vi "FilePath.vi"(8 "error in":errorcluster) -> (0 "error out":errorcluster, 3 "File path":path)   [LabVIEW 2016]
doc: "This SubVI designed for create filepath\nwith specific filename for saving picture\nto local disc. File name generate following\nto current date/time"
panel:
  # "This SubVI designed for create filepath\nwith specific filename for saving picture\nto local disc. File name generate following\nto current date/time"
  # "Outputs"
  # "Inputs"
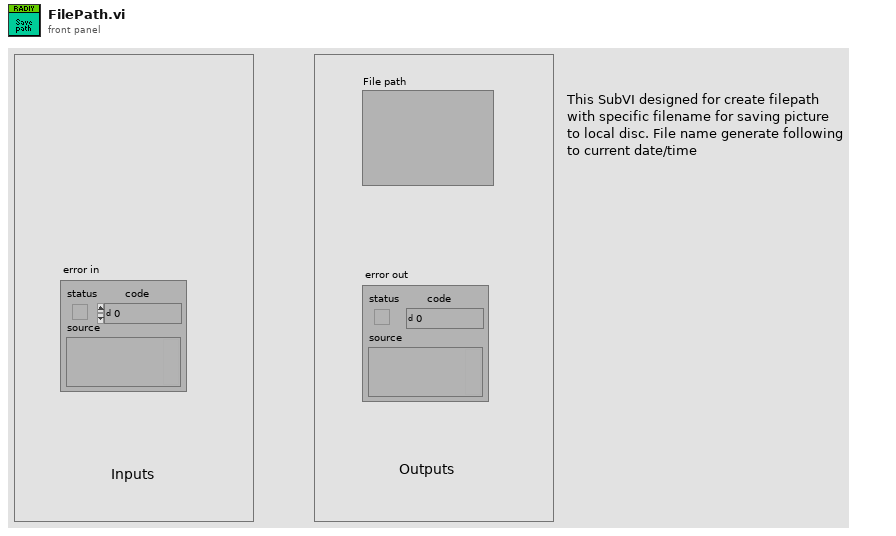
[diagram p1: front panel]
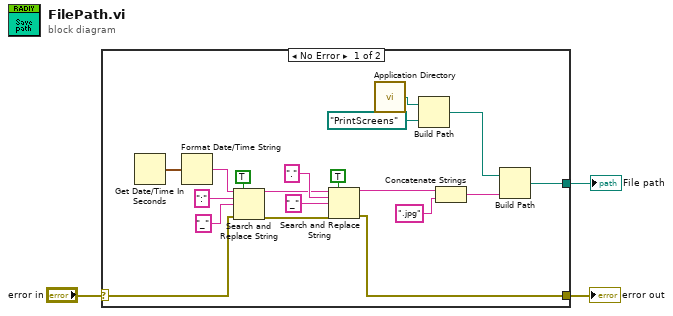
[diagram p0: block diagram]
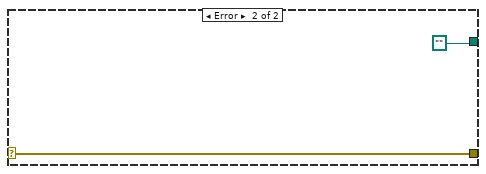
[diagram p2: hidden frame]
diagram:
  n1 = case shown="No Error" "error in" {
    selector: "error in" -> [w19 w24]
    tunnel: [w9 w24] -> w2
    tunnel: [w20 path ""] -> w1
    frame No Error {
      n2 = Get Date/Time In Seconds() -> (seconds since 1Jan1904=w18:timestamp)
      n3 = Format Date/Time String(seconds (now)=w18) -> (date/time string=w11:string)  [unwired: 2 in]
      n4 = Search and Replace String(replace all?=TRUE ("replace all? (F)"), input string=w11, search string=":", replace string="_" ("string"), error in=w19) -> (result string=w13:string, error out=w12:errorcluster)  [unwired: 3 in, 2 out]
      n5 = Search and Replace String(replace all?=TRUE ("replace all? (F)"), input string=w13, search string=".", replace string="_" ("string"), error in=w12) -> (result string=w8:string, error out=w9:errorcluster)  [unwired: 3 in, 2 out]
      n6 = call <vilib>:"Application Directory.vi"() -> ("Application Directory"=w4:path)
      n7 = Build Path(base path=w4, name or relative path=path "PrintScreens") -> (appended path=w5:path)
      n8 = Concatenate Strings(w8, ".jpg" ("replace string (\"\")")) -> (w7:string)
      n9 = Build Path(base path=w5, name or relative path=w7) -> (appended path=w20:path)
    }
    frame Error {
    }
  }
  "error out" <- w2
  "File path" <- w1
